vi "UploadFileWebService.vi"() -> ()   [LabVIEW 2021]
uses:
  <vilib>/httpClient/MultipartData.ctl
  <vilib>/httpClient/POSTFile.vi
  <vilib>/httpClient/LabVIEWHTTPClient.lvlib
panel:
  out "body":string
  out "headers":string
  out "error out":errorcluster
  in  "UploadButton":bool
  in  "StopButton":bool
  in  "File Path":path
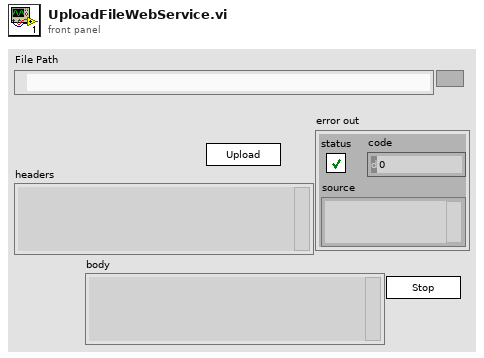
[diagram p1: front panel]
types:
  T1 = typedef "LabVIEWHTTPClient.lvlib/ClientHandle.ctl" = refnum<k1>
  T2 = typedef "LabVIEWHTTPClient.lvlib/MultipartData.ctl" = cluster{"Name":string, "Value":string, "File":path, "Filename":string, "MIME type":string}
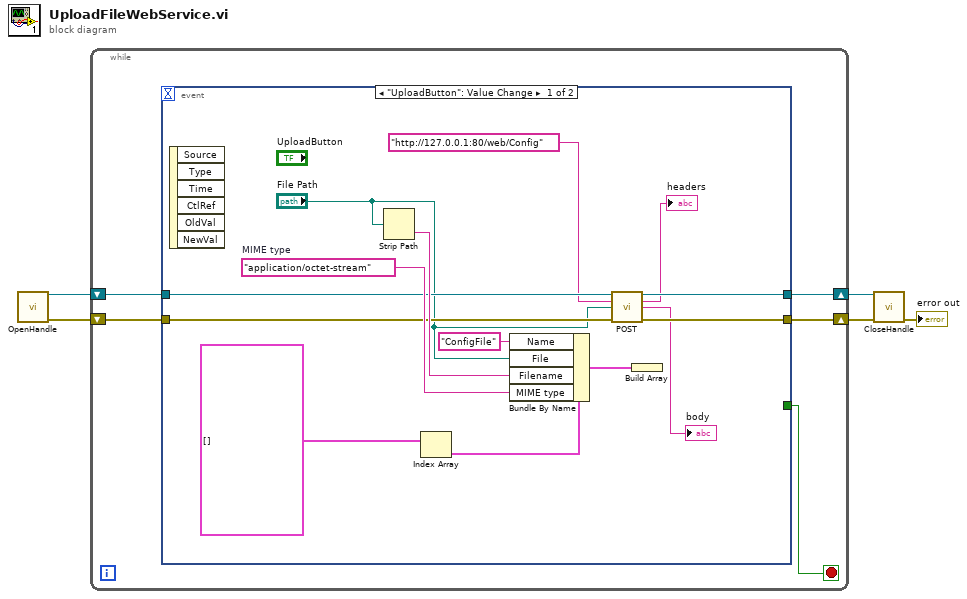
[diagram p0: block diagram]
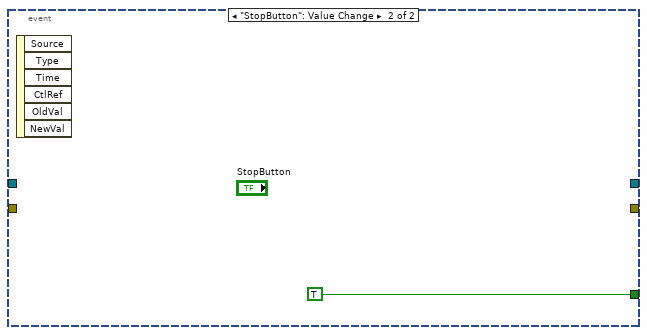
[diagram p2: hidden frame]
diagram:
  n1 = call <vilib>:"OpenHandle.vi"() -> ("client handle out"=w5:T1, "error out"=w3:errorcluster)  [unwired: 14 in]
  n2 = while {
    shift-right: [w9] -> w4
    shift-left: w5 -> [w10]
    shift-right: [w7] -> w2
    shift-left: w3 -> [w8]
    stop <- w6 stop-if-true
    n3 = event shown="[0] \"UploadButton\": Value Change" {
      selector: _ -> [_ _]
      dyn-events: _ -> [_ _]
      timeout: _ -> [_ _]
      tunnel: w10 -> [w18 _]
      tunnel: [w17 _] -> w9
      tunnel: w8 -> [w15 _]
      tunnel: [w16 _] -> w7
      tunnel: [_ TRUE] -> w6
      event "UploadButton": Value Change {
        w22 = "application/octet-stream"  # MIME type
        n4 = event-data() -> ()  [unwired: 1 in, 6 out]
        n5 = Strip Path(path="File Path") -> (name=w21:string)  [unwired: 1 out]
        n6 = Index Array(array=T2[] [] ("data")) -> (element=w20:T2)  [unwired: 1 in]
        n7 = Bundle By Name(cluster=w20, "Name"="ConfigFile", "File"="File Path", "Filename"=w21, "MIME type"=w22) -> (w24:T2)
        n8 = call-poly <vilib>:"POST.vi"("client handle"=w18, "url"="http://127.0.0.1:80/web/Config", "file"="File Path", "error in (no error)"=w15) -> ("client handle out"=w17:T1, "headers"=→"headers":string, "body"=→"body":string, "error out"=w16:errorcluster)  [unwired: 8 in]
        n9 = Build Array(w24) -> ()  [unwired: 1 out]
      }
      event "StopButton": Value Change {
        n10 = event-data() -> ()  [unwired: 1 in, 6 out]
      }
    }
  }
  n11 = call <vilib>:"CloseHandle.vi"("client handle"=w4, "error in (no error)"=w2) -> ("error out"=→"error out":errorcluster)  [unwired: 13 in]
